vi "criteria string.vi"(7 "Sequence step config":T1, 9 "Finnished(F)":bool, 12 "User input":dbl) -> (8 "Full criteria string":string, 10 "Actino string":string)   [LabVIEW 2011]
uses:
  Sequence steps config..ctl
  Single criteria cluster.ctl
  Criteria types.ctl
  Boolean operation.ctl
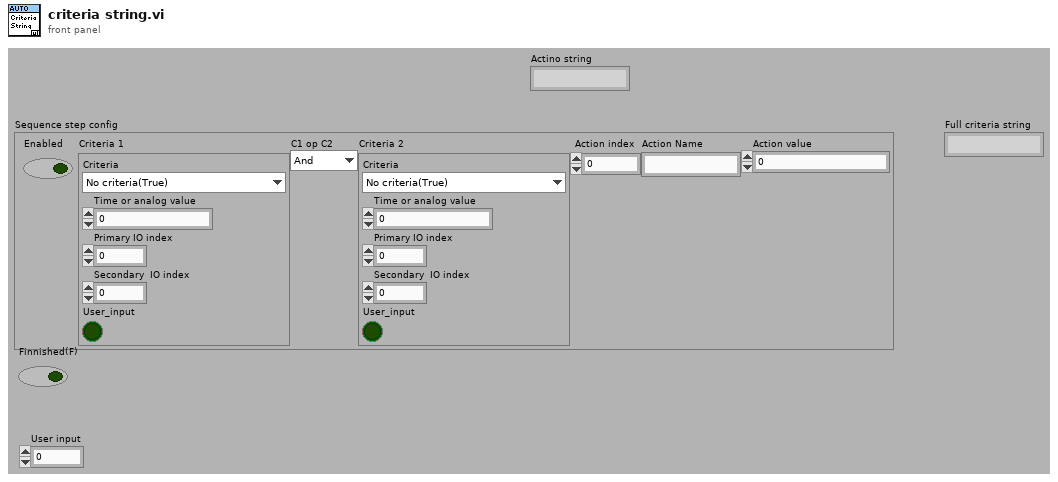
[diagram p1: front panel]
types:
  T1 = typedef "Sequence steps config..ctl" = cluster{"Enabled":bool, "Criteria 1":T2, "C1 op C2":T4, "Criteria 2":T2, "Action index":i32, "Action Name":string, "Action value":dbl}
  T2 = typedef "Single criteria cluster.ctl" = cluster{"Criteria":T3, "Time or analog value":dbl, "Primary IO index":i32, "Secondary  IO index":i32, "User_input":bool}
  T3 = typedef "Criteria types.ctl" = enum16{"No criteria(True)", "Time(s)", "Analog IO over", "Analog IO over or equal", "Analog IO under", "Analog IO under or equal", "Analog IO 1 minus Analog IO 2 over", "Digital IO True", "Digital IO False", "Operator approval"}
  T4 = typedef "Boolean operation.ctl" = enum16{"And", "Or", "Xor", "Nand", "Nor", "Nxor", "Implies"}
  T5 = typedef "Action colleciton cluster.ctl" = cluster{"common":T6, "Action type":T8, "General command":T9, "PCP command":T10, "Tool command":T11}
  T6 = typedef "Action common elements.ctl" = cluster{"Name":string, "Adjuster type":T7, "Adjuster double default value":dbl}
  T7 = typedef "Action adjuster type.ctl" = enum16{"Non", "Double"}
  T8 = typedef "Action type.ctl" = enum16{"General", "PCP command", "Tool command"}
  T9 = typedef "General command list.ctl" = enum16{"No action"}
  T10 = typedef "PCP High Level Commands.ctl" = enum16{"HVPSU HV ON", "HVPSU HV OFF", "PCP PC", "PCP Local", "Update Motor Voltage", "Update Cable Resistance", "Final Motor Voltage", "Final Resistance"}
  T11 = typedef "Tool specific commands.ctl" = enum16{"controller relay 1 on", "controller relay 1 off", "controller relay 2 on", "controller relay 2 off", "Solonoid 1 (master) on", "Solonoid 1 (master) off", "Solonoid 2 (Stroker) on", "Solonoid 2 (Stroker) off", "Solonoid 3 (Anchor) on", "Solonoid 3 (Anchor) off", "Controller relay 1 & 2 on", "Controller relay 1 & 2 off", "Controller relay 1 on, 2 off", "Controller relay 1 off, 2 on", "STROKER tool: Stop Force Mon", "High-G Stop", "High-G Get data", "High-G Stop Get data", "STROKER tool: Stroke out", "STROKER tool: Stroke in", "STROKER tool: Stroke stop", "STROKER tool: Stroke go to", "STROKER tool: Stop Homing", "STROKER tool: Start Force Mon dir in", "STROKER tool: Start Force Mon dir out", "Controller STOP"}
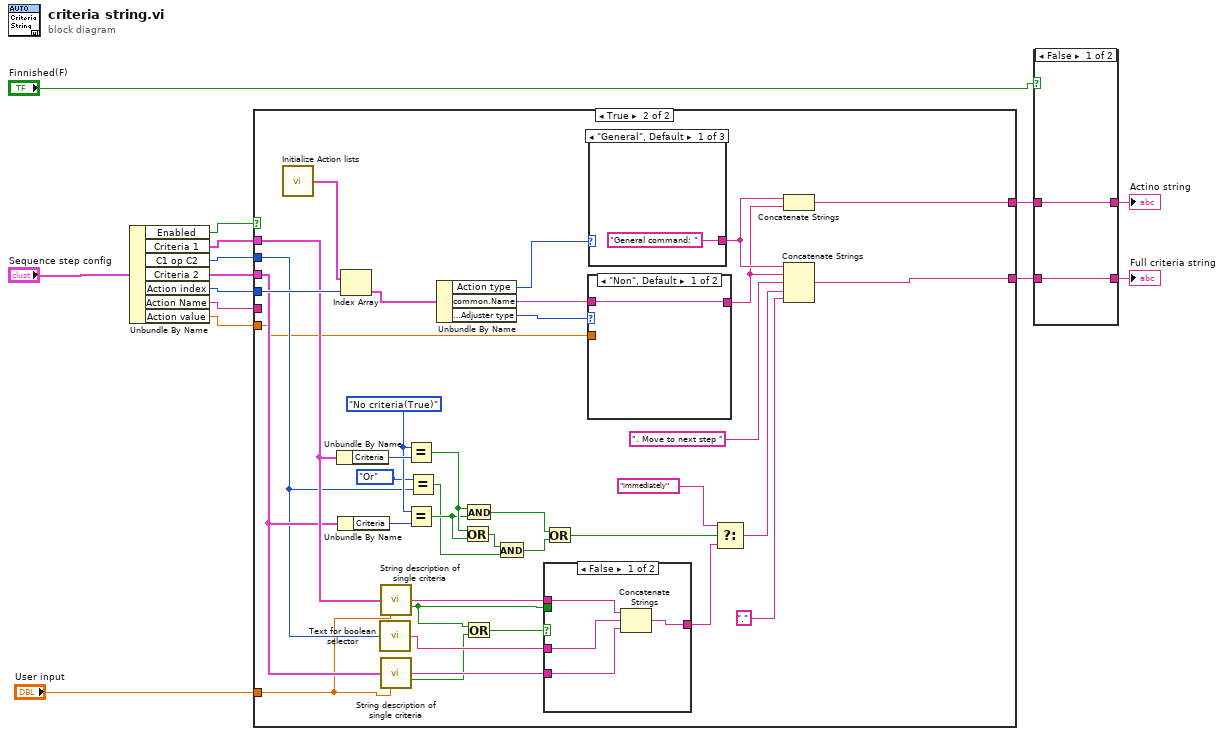
[diagram p0: block diagram]
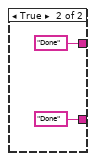
[diagram p2: hidden frame]
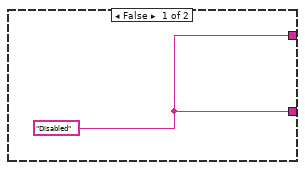
[diagram p3: hidden frame]
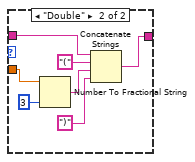
[diagram p6: hidden frame]
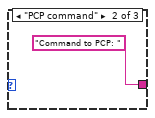
[diagram p7: hidden frame]
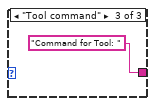
[diagram p8: hidden frame]
diagram:
  n1 = Unbundle By Name("Sequence step config") -> ("Enabled"=w9:bool, "Criteria 1"=w12:T2, "C1 op C2"=w14:T4, "Criteria 2"=w13:T2, "Action index"=w11:i32, "Action Name"=w10:string, "Action value"=w7:dbl)
  n2 = case shown="True" w9 {
    tunnel: w10 -> [_ _]
    tunnel: w11 -> [_ w51]
    tunnel: w12 -> [_ w31]
    tunnel: w13 -> [_ w30]
    tunnel: w14 -> [_ w27]
    tunnel: [w15 w32] -> w2
    tunnel: w7 -> [_ w20]
    tunnel: [w15 w17] -> w4
    tunnel: "User input" -> [_ w16]
    frame False {
      w15 = "Disabled"
    }
    frame True {
      w43 = Criteria_types."No criteria(True)" ("x")
      n3 = call "Initialize Action lists.vi"() -> ("Actions"=w52:T5[])  [unwired: 13 in, 2 out]
      n4 = Unbundle By Name(w31) -> ("Criteria"=w45:T3)
      n5 = Unbundle By Name(w30) -> ("Criteria"=w44:T3)
      n6 = Index Array(array=w52, index=w51) -> (element=w50:T5)
      n7 = call "Text for boolean selector.vi"("C1 op C2"=w27) -> ("String"=w26:string)  [unwired: 14 in]
      n8 = call "String description of single criteria.vi"("Criteria"=w31, "User input"=w16) -> ("String"=w29:string, "Immediate"=w23:bool)  [unwired: 12 in]
      n9 = call "String description of single criteria.vi"("Criteria"=w30, "User input"=w16) -> ("String"=w28:string, "Immediate"=w25:bool)  [unwired: 12 in]
      n10 = Equal?(x=w43, y=w45) -> (x = y?=w41:bool)
      n11 = Equal?(x=w43, y=w44) -> (x = y?=w40:bool)
      n12 = Equal?(x=Boolean_operation."Or", y=w27) -> (x = y?=w38:bool)
      n13 = Unbundle By Name(w50) -> ("Action type"=w49:T8, "common.Name"=w47:string, "common.Adjuster type"=w48:T7)
      n14 = Or(x=w41, y=w40) -> (x .or. y?=w39:bool)
      n15 = And(x=w41, y=w40) -> (x .and. y?=w36:bool)
      n16 = Or(x=w23, y=w25) -> (x .or. y?=w24:bool)
      n17 = And(x=w39, y=w38) -> (x .and. y?=w37:bool)
      n18 = case shown="False" w24 {
        tunnel: w29 -> [w56 w59]
        tunnel: w28 -> [w54 w58]
        tunnel: w26 -> [w55 _]
        tunnel: [w53 w57] -> w22
        tunnel: w23 -> [_ w60]
        frame False {
          n19 = Concatenate Strings(w56, w55, w54) -> (w53:string)
        }
        frame True {
          n20 = case shown="False" w60 {
            tunnel: w59 -> [w61 _]
            tunnel: w58 -> [_ w62]
            tunnel: [w61 w62] -> w57
            frame False {
            }
            frame True {
            }
          }
        }
      }
      n21 = Or(x=w36, y=w37) -> (x .or. y?=w35:bool)
      n22 = case shown="\"Non\", Default" w48 {
        tunnel: w47 -> [w63 w69]
        tunnel: w20 -> [_ w70]
        tunnel: [w63 w65] -> w18
        frame "Non", Default {
        }
        frame "Double" {
          n23 = Number To Fractional String(number=w70, precision (6)=i16 3) -> (F-format string=w68:string)  [unwired: 2 in]
          n24 = Concatenate Strings(w69, "(" ("string"), w68, ")" ("string")) -> (w65:string)
        }
      }
      n25 = case shown="\"General\", Default" w49 {
        tunnel: ["General command: " "Command to PCP: " "Command for Tool: "] -> w19
        frame "General", Default {
        }
        frame "PCP command" {
        }
        frame "Tool command" {
        }
      }
      n26 = Select(t="immediately" ("string"), s=w35, f=w22) -> (s? t:f=w33:string)
      n27 = Concatenate Strings(w19, w18) -> (w17:string)
      n28 = Concatenate Strings(w19, w18, ". Move to next step " ("string"), w33, "." ("string")) -> (w32:string)
    }
  }
  n29 = case shown="False" "Finnished(F)" {
    tunnel: [w75 "Done"] -> w5
    tunnel: w4 -> [w75 _]
    tunnel: [w74 "Done"] -> w3
    tunnel: w2 -> [w74 _]
    frame False {
    }
    frame True {
    }
  }
  "Full criteria string" <- w3
  "Actino string" <- w5
